vi "Globals - Streams.vi"() -> ()   [LabVIEW 2013]
panel:
  in  "RT Message Stream":refnum<k21>
  in  "UI Command Stream":refnum<k21>
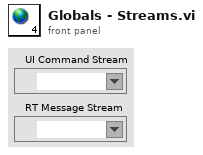
[diagram p1: front panel]
diagram:
